vi "transAndPhaseManager.vi"(0 "Trans in":dbl(slide) scale=0.0..100.0, 2 "Trans mod":dbl=2.0, 9 "Phase in":dbl(slide) scale=0.0..360.0, 13 "Phase mod":dbl=15.0) -> (4 "Trans %":dbl=100.0, 6 "Intensity":dbl=100.0, 8 "T gl":dbl, 10 "Phase Deg":dbl, 15 "Phase Rad":dbl)   [LabVIEW 2023]
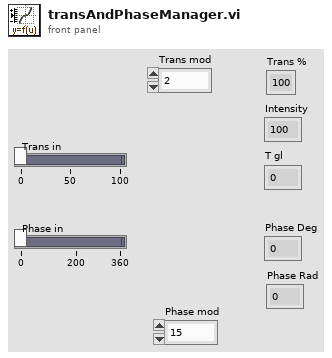
[diagram p1: front panel]
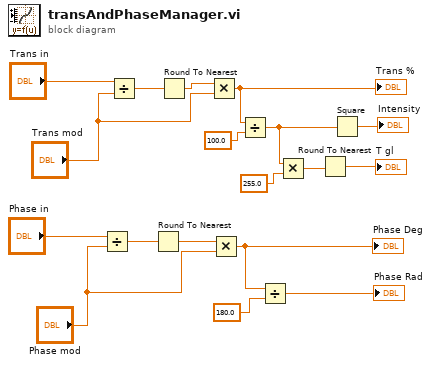
[diagram p0: block diagram]
diagram:
  n1 = Divide(x="Phase in", y="Phase mod") -> (x/y=w12:dbl)
  n2 = Divide(x="Trans in", y="Trans mod") -> (x/y=w17:dbl)
  n3 = Round To Nearest(number=w12) -> (nearest integer value=w11:dbl)
  n4 = Round To Nearest(number=w17) -> (nearest integer value=w16:dbl)
  n5 = Multiply(x=w16, y="Trans mod") -> (x*y=w4:dbl)
  "Trans %" <- w4
  n6 = Multiply(x=w11, y="Phase mod") -> (x*y=w10:dbl)
  "Phase Deg" <- w10
  n7 = Divide(x=w4, y=100.0) -> (x/y=w3:dbl)
  n8 = Divide(x=w10, y=180.0) -> (x/y=→"Phase Rad":dbl)
  n9 = Multiply(x=w3, y=255.0) -> (x*y=w2:dbl)
  n10 = Round To Nearest(number=w2) -> (nearest integer value=→"T gl":dbl)
  n11 = Square(x=w3) -> (x^2=→"Intensity":dbl)
